vi "ActionVIOnCompile.vi"(8 "error in (no error)":errorcluster, 11 "Device Item Ref in":T1 format="%.0x") -> (0 "error out":errorcluster)   [LabVIEW 2021, in "Large Number Operation System Explorer.lvlib"]
uses:
  Large Number Operation System Explorer.lvlib
  <vilib>/NI VeriStand/Custom Device API/Custom Device Item Ref.ctl
  Shared/Compiled.Settings.ctl
  <vilib>/NI VeriStand/Custom Device API/Get Item Property (U16).vi
  <vilib>/NI VeriStand/Custom Device API/Get Item Property (String).vi
  <vilib>/NI VeriStand/Custom Device Tools/Custom Device Utility Library/NI VeriStand - Search for Item by Name.vi
  <vilib>/NI VeriStand/Custom Device API/Set Item Property (Variant).vi
  <vilib>/NI VeriStand/Custom Device Tools/Custom Device Utility Library/Custom Device Utility Library.lvlib
  <vilib>/NI VeriStand/Custom Device API/Custom Device API.lvlib
  <vilib>/NI/NIVS Inline Async API/_Data Access System Explorer/Data Access System Explorer.lvlib
  Shared/Large Number Operation Shared.lvlib
  Shared/Constants.vi
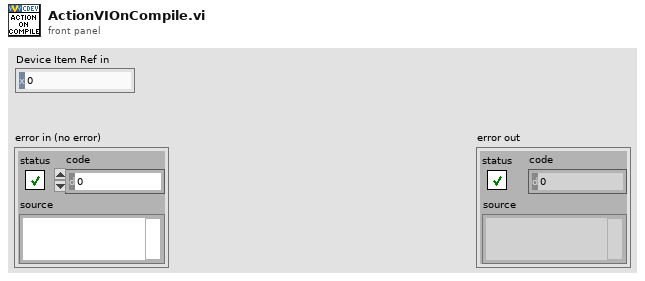
[diagram p1: front panel]
types:
  T1 = typedef "Custom Device API.lvlib/Custom Device Item Ref.ctl" = u64
  T2 = cluster{"Name":string, "Type":enum16{"Output/Write", "Input/Read", "Input/ReadWrite"}, "VS Refs":T1[]}
  T3 = enum16{"Output/Write", "Input/Read", "Input/ReadWrite"}
  T4 = typedef "Large Number Operation Shared.lvlib/Compiled.Settings.ctl" = cluster{"Name":string, "Async Init Timeout":u16, "Address":string}
  T5 = typedef "Custom Device API.lvlib/Custom Device Item Info.ctl" = cluster{"Name":string, "Is Channel":bool, "GUID":string, "Is Waveform":bool}
  T6 = cluster{"Name":string, "Type":enum16{"Output/Write", "Input/Read", "Input/ReadWrite"}, "VS Refs":T1[]}[]
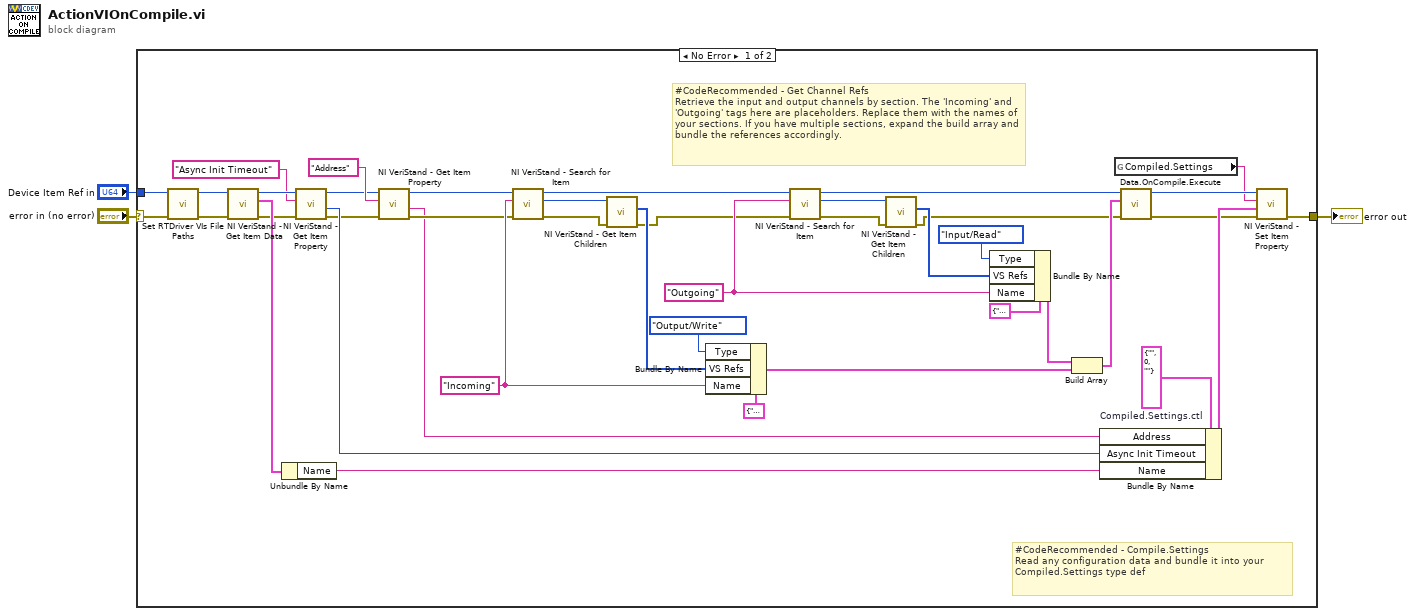
[diagram p0: block diagram]
diagram:
  n1 = case shown="No Error" "error in (no error)" {
    selector: "error in (no error)" -> [w13 w45]
    tunnel: [w39 w45] -> w2
    tunnel: "Device Item Ref in" -> [w14 _]
    frame No Error {
      w19 = T4 {"Name"="", "Async Init Timeout"=0, "Address"=""}  # Compiled.Settings.ctl
      w34 = "Outgoing" ("Item Name")
      w36 = "Incoming" ("Item Name")
      # "#CodeRecommended - Get Channel Refs\nRetrieve the input and output channels by section. The 'Incoming' and 'Outgoing' tags here are placeholders. Replace them with the names of your sections. If you have multiple sections, expand the build array and bundle the references accordingly."
      # "#CodeRecommended - Compile.Settings\nRead any configuration data and bundle it into your Compiled.Settings type def"
      n2 = call "Set RTDriver VIs File Paths.vi"("error in (no error)"=w13, "Item Ref in"=w14) -> ("error out"=w11:errorcluster, "Item Ref out"=w12:T1)  [unwired: 8 in]
      n3 = call <vilib>:"NI VeriStand - Get Item Data.vi"("error in (no error)"=w11, "Item Ref in"=w12) -> ("error out"=w18:errorcluster, "Item Info"=w38:T5, "Item Ref out"=w17:T1)  [unwired: 6 in, 1 out]
      n4 = Unbundle By Name(w38) -> ("Name"=w37:string)
      n5 = call-poly <vilib>:"NI VeriStand - Get Item Property.vi"("error in (no error)"=w18, "Property Name"="Async Init Timeout", "Item Ref in"=w17) -> ("error out"=w6:errorcluster, "Value"=w15:u16, "Item Ref out"=w9:T1)  [unwired: 5 in, 1 out]
      n6 = call-poly <vilib>:"NI VeriStand - Get Item Property.vi"("error in (no error)"=w6, "Property Name"="Address", "Item Ref in"=w9) -> ("error out"=w7:errorcluster, "Value"=w5:string, "Item Ref out"=w8:T1)  [unwired: 5 in, 1 out]
      n7 = call-poly <vilib>:"NI VeriStand - Search for Item.vi"("error in"=w7, "Item Name"=w36, "Section Ref in"=w8) -> ("error out"=w44:errorcluster, "Item Ref"=w43:T1, "Section Ref out"=w23:T1)  [unwired: 5 in, 1 out]
      n8 = call <vilib>:"NI VeriStand - Get Item Children.vi"("error in (no error)"=w44, "Item Ref in"=w43) -> ("error out"=w22:errorcluster, "Child Refs"=w35:T1[])  [unwired: 6 in, 2 out]
      n9 = Bundle By Name(cluster=T2 {"Name"="", "Type"=enum."Output/Write", "VS Refs"=[]} ("Group"), "Type"=T3."Output/Write", "VS Refs"=w35, "Name"=w36) -> (w26:T2)
      n10 = call-poly <vilib>:"NI VeriStand - Search for Item.vi"("error in"=w22, "Item Name"=w34, "Section Ref in"=w23) -> ("error out"=w41:errorcluster, "Item Ref"=w42:T1, "Section Ref out"=w24:T1)  [unwired: 5 in, 1 out]
      n11 = call <vilib>:"NI VeriStand - Get Item Children.vi"("error in (no error)"=w41, "Item Ref in"=w42) -> ("error out"=w25:errorcluster, "Child Refs"=w30:T1[])  [unwired: 6 in, 2 out]
      n12 = Bundle By Name(cluster=T2 {"Name"="", "Type"=enum."Output/Write", "VS Refs"=[]} ("Group"), "Type"=T3."Input/Read", "VS Refs"=w30, "Name"=w34) -> (w32:T2)
      n13 = Build Array(w32, w26) -> (w29:T6)
      n14 = Bundle By Name(cluster=w19, "Address"=w5, "Async Init Timeout"=w15, "Name"=w37) -> (w40:T4)
      n15 = global read "Constants.vi" "Compiled.Settings"() -> (w4:string)
      n16 = call <vilib>:"Data.OnCompile.Execute.vi"("error in"=w25, "VS Ref Groups"=w29, "Custom Device Ref"=w24) -> ("error out"=w21:errorcluster, "Custom Device Ref"=w20:T1)  [unwired: 7 in]
      n17 = call-poly <vilib>:"NI VeriStand - Set Item Property.vi"("error in (no error)"=w21, "Value"=w40, "Property Name"=w4, "Item Ref in"=w20) -> ("error out"=w39:errorcluster)  [unwired: 5 in, 2 out]
    }
    frame Error {
    }
  }
  "error out" <- w2
